vi "AssertValueByArrayName.vi"(0 "VI Reference In":refnum<vi>, 1 "Test Label":string, 2 "delimiter (>>)":string=">>", 3 "Assert Only? (F)":bool, 5 "Control Path":string, 7 "Focus Item Names":string[](array[string]), 11 "Error In":errorcluster, 12 "Assert Interval(10 ms)":u32=10, 13 "Timeout(5 sec)":dbl=5.0) -> (4 "VI Reference Out":refnum<vi>, 6 "Asserted Value":string[](array[string]), 15 "Error Out":errorcluster)   [LabVIEW 2016, in "Drona.lvlib" / "AssertControlValue.lvlib" / "AssertMCListbox.lvlib"]
doc: "Asserts if the focus item first column names of multi-select listbox control are equal.\n\nThe input control name is given as a string, incase of the path, use delimiters in between the path.\nThis VI gets the control value until the value is equal to the input value."
uses:
  AssertMCListbox.lvlib
  Get/GetControlRef/GetControlRefByPath.vi
  <userlib>/_OpenG.lib/array/array.llb/Index 1D Array Elements (String)__ogtk.vi
  <vilib>/addons/_JKI Toolkits/Caraya/classes/Assert/Assert Equal Value_Variant.vi
  <vilib>/Utility/error.llb/Error Cluster From Error Code.vi
  <vilib>/ErrorRing/Error Ring.xnode
  <vilib>/addons/_JKI Toolkits/Caraya/classes/Assert/Assert.lvclass
  Get/GetControlRef/GetControlRef.lvlib
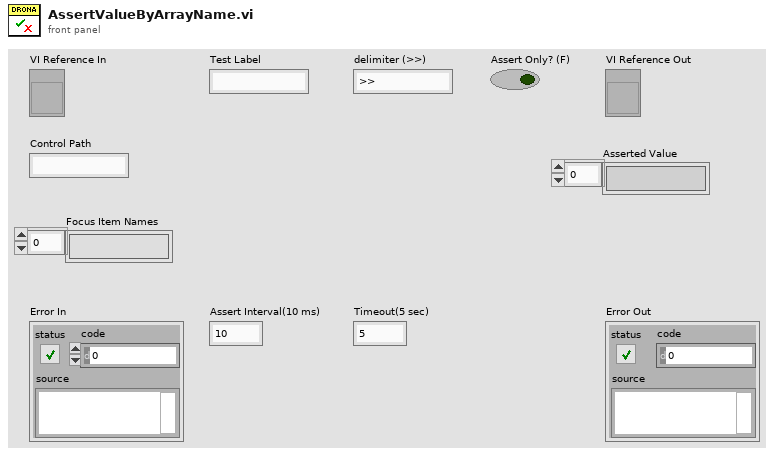
[diagram p1: front panel]
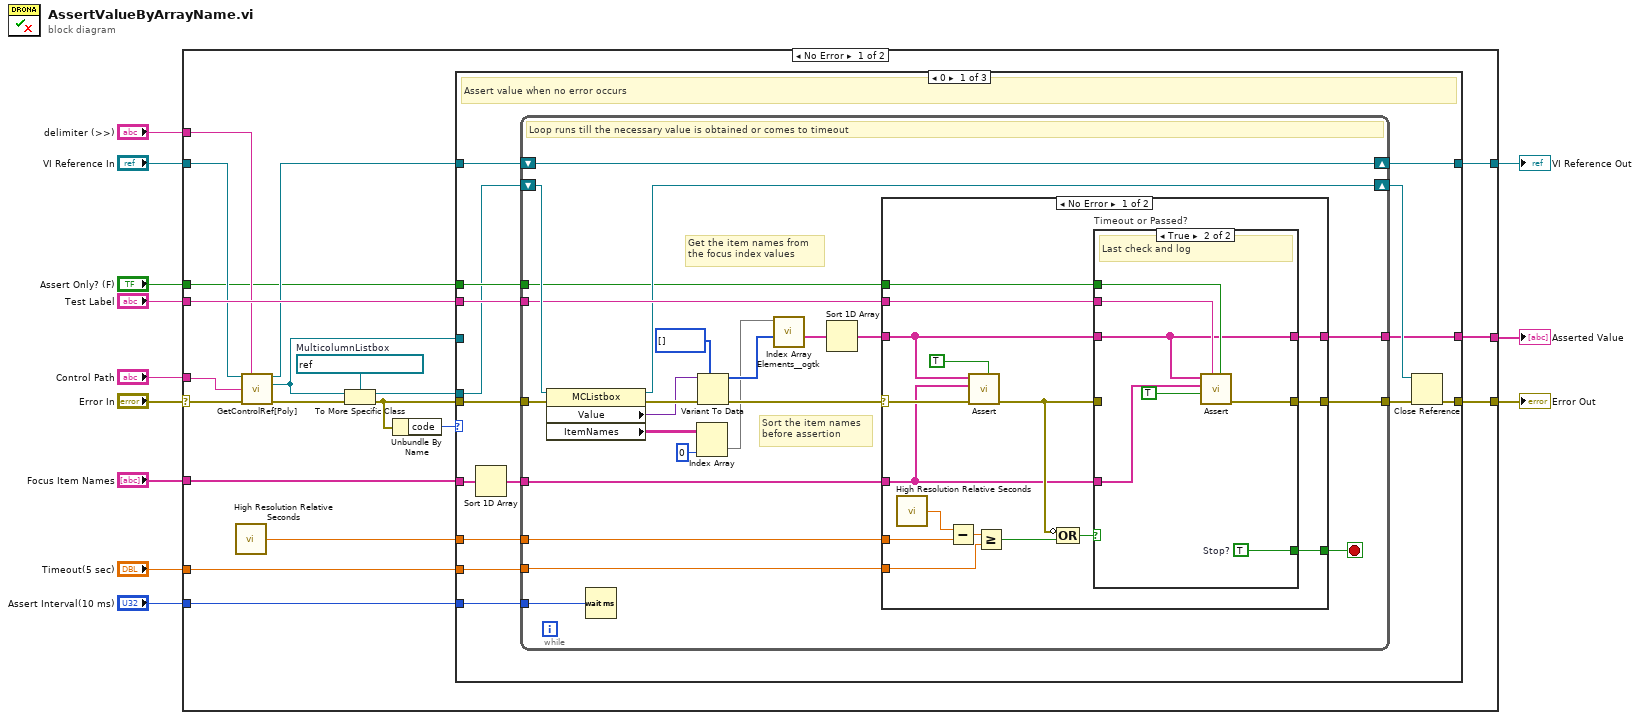
[diagram p0: block diagram]
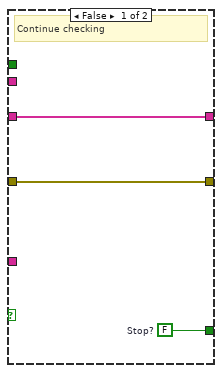
[diagram p2: hidden frame]
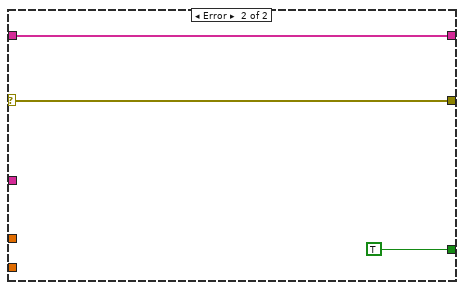
[diagram p3: hidden frame]
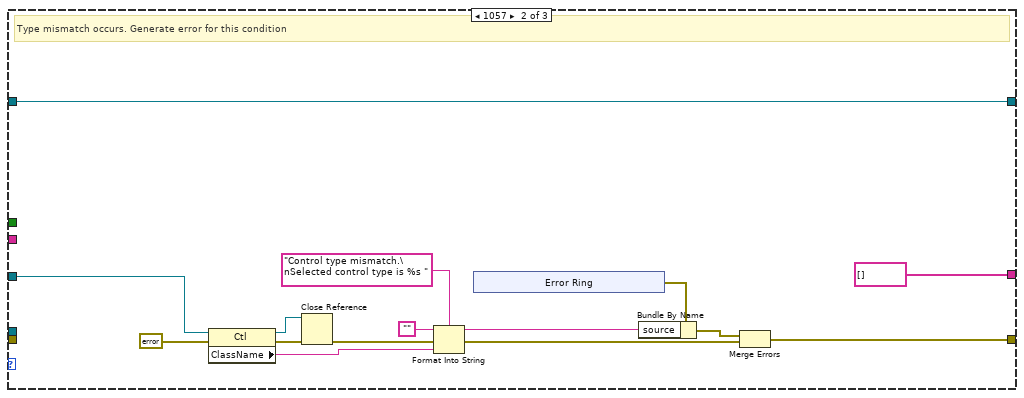
[diagram p4: hidden frame]
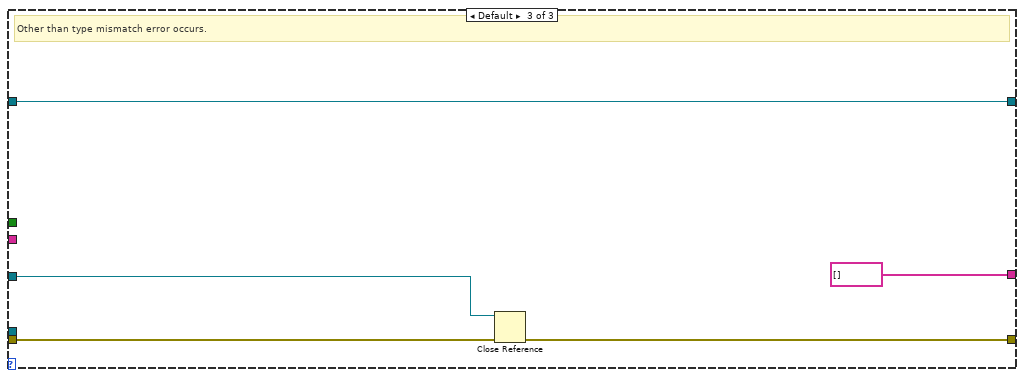
[diagram p5: hidden frame]
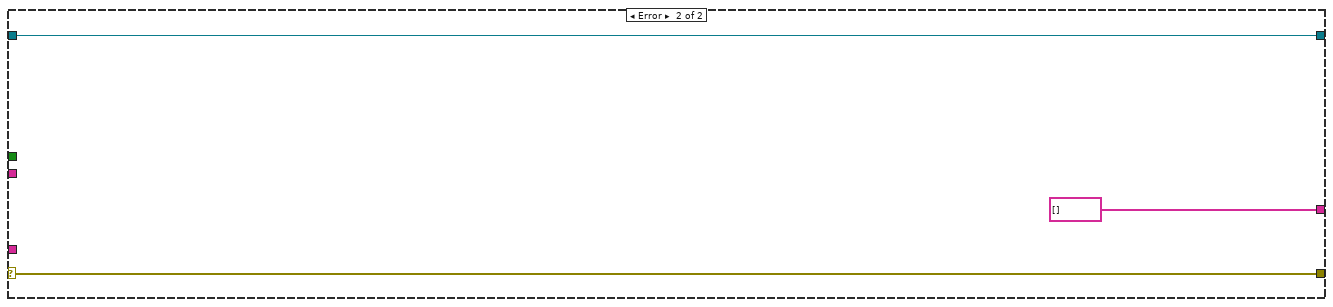
[diagram p6: hidden frame]
diagram:
  n1 = case shown="No Error" "Error In" {
    selector: "Error In" -> [w28 w127]
    tunnel: "Timeout(5 sec)" -> [w32 _]
    tunnel: [w31 w126] -> w11
    tunnel: [w22 w127] -> w10
    tunnel: "Assert Interval(10 ms)" -> [w30 _]
    tunnel: "Test Label" -> [w29 _]
    tunnel: "VI Reference In" -> [w27 w126]
    tunnel: "Control Path" -> [w26 _]
    tunnel: "delimiter (>>)" -> [w21 _]
    tunnel: "Assert Only? (F)" -> [w20 _]
    tunnel: [w19 string[] []] -> w2
    tunnel: "Focus Item Names" -> [w16 _]
    frame No Error {
      w18 = refnum<vi> refnum  # MulticolumnListbox
      n2 = call <vilib>:"High Resolution Relative Seconds.vi"() -> ("relative seconds"=w25:dbl)
      n3 = call-poly "GetControlRef[Poly].vi"("VI Reference In"=w27, "delimiter (>>)"=w21, "Control Path"=w26, "error In"=w28) -> ("VI Reference Out"=w23:refnum<vi>, "Ctl Refnum"=w13:refnum<vi>, "error out"=w24:errorcluster)  [unwired: 9 in]
      n4 = To More Specific Class(target class=w18, reference=w13, error in=w24) -> (specific class reference=w17:refnum<vi>, error out=w15:errorcluster)
      n5 = Unbundle By Name(w15) -> ("code"=w14:i32)
      n6 = case shown="0" w14 {
        tunnel: w32 -> [w47 _ _]
        tunnel: [w46 w100 w123] -> w31
        tunnel: w30 -> [w44 _ _]
        tunnel: w29 -> [w43 _ _]
        tunnel: w25 -> [w42 _ _]
        tunnel: w23 -> [w41 w100 w123]
        tunnel: [w40 w103 w121] -> w22
        tunnel: w20 -> [w38 _ _]
        tunnel: [w33 string[] [] string[] []] -> w19
        tunnel: w15 -> [w37 _ w124]
        tunnel: w17 -> [w36 _ _]
        tunnel: w16 -> [w35 _ _]
        tunnel: w13 -> [_ w102 w120]
        frame 0 {
          # "Assert value when no error occurs"
          n7 = Sort 1D Array(array=w35) -> (sorted array=w34:string[])
          n8 = while {
            tunnel: w47 -> [w69]
            tunnel: w42 -> [w70]
            tunnel: w37 -> [w64]
            tunnel: [w67] -> w45
            tunnel: w44 -> [w65]
            tunnel: w43 -> [w61]
            shift-right: [w62] -> w46
            shift-left: w41 -> [w62]
            shift-right: [w60] -> w39
            shift-left: w36 -> [w63]
            tunnel: w38 -> [w59]
            tunnel: [w58] -> w33
            tunnel: w34 -> [w54]
            stop <- w68 stop-if-true
            # "Sort the item names \nbefore assertion"
            # "Get the item names from \nthe focus index values"
            # "Loop runs till the necessary value is obtained or comes to timeout"
            n9 = property on="Property Node" class="MCListbox"(reference=w63, error in=w64) -> (reference out=w60:refnum<vi>, error out=w66:errorcluster, "Value"=w56:variant, "ItemNames"=w50:string[][])
            n10 = Wait (ms)(milliseconds to wait=w65) -> ()  [unwired: 1 out]
            n11 = Index Array(array=w50, index (col)=0 ("disabled index (col)")) -> (element=w48:string[])  [unwired: 1 in]
            n12 = Variant To Data(error in=w66, type=i32[] [], Variant=w56) -> (data=w52:i32[], error out=w57:errorcluster)
            n13 = call-poly <userlib>:"Index Array Elements__ogtk.vi"("indices"=w52, "array"=w48) -> ("elements"=w51:string[])  [unwired: 9 in]
            n14 = Sort 1D Array(array=w51) -> (sorted array=w53:string[])
            n15 = case shown="No Error" w57 {
              selector: w57 -> [w82 w99]
              tunnel: w70 -> [w86 _]
              tunnel: w69 -> [w83 _]
              tunnel: [w73 TRUE] -> w68
              tunnel: [w74 w99] -> w67
              tunnel: w54 -> [w75 _]
              tunnel: w53 -> [w76 w97]
              tunnel: w61 -> [w81 _]
              tunnel: w59 -> [w72 _]
              tunnel: [w71 w97] -> w58
              frame No Error {
                n16 = call <vilib>:"High Resolution Relative Seconds.vi"() -> ("relative seconds"=w85:dbl)
                n17 = Subtract(x=w85, y=w86) -> (x-y=w84:dbl)
                n18 = call-poly <vilib>:"Assert.vi"("Assert Only? (F)"=TRUE, "error in (no error)"=w82, "Y"=w75, "X"=w76) -> ("error out"=w79:errorcluster)  [unwired: 6 in, 1 out]
                n19 = Greater Or Equal?(x=w84, y=w83) -> (x >= y?=w80:bool)
                n20 = Compound Arithmetic op=OR(invert w79, w80) -> (w78:bool)
                n21 = case "Timeout or Passed?" shown="True" w78 {
                  tunnel: w79 -> [w89 _]
                  tunnel: w75 -> [_ w91]
                  tunnel: w76 -> [w87 w92]
                  tunnel: w81 -> [_ w96]
                  tunnel: [w89 w95] -> w74
                  tunnel: [w88 w94] -> w73
                  tunnel: w72 -> [_ w93]
                  tunnel: [w87 w92] -> w71
                  frame False {
                    w88 = FALSE  # Stop?
                    # "Continue checking"
                  }
                  frame True {
                    w94 = TRUE  # Stop?
                    # "Last check and log"
                    n22 = call-poly <vilib>:"Assert.vi"("Assert Only? (F)"=w93, "Label"=w96, "Register with caller test (F)"=TRUE, "Y"=w91, "X"=w92) -> ("error out"=w95:errorcluster)  [unwired: 5 in, 1 out]
                  }
                }
              }
              frame Error {
              }
            }
          }
          n23 = Close Reference(reference=w39, error in (no error)=w45) -> (error out=w40:errorcluster)
        }
        frame 1057 {
          # "Type mismatch occurs. Generate error for this condition"
          n24 = property class="Ctl"(reference=w102, error in=errorcluster {"status"=FALSE, "code"=0, "source"=""} ("error out")) -> (reference out=w104:refnum<vi>, error out=w114:errorcluster, "ClassName"=w111:string)
          n25 = Close Reference(reference=w104, error in (no error)=w114) -> (error out=w105:errorcluster)
          n26 = Format Into String(format string="Control type mismatch.\nSelected control type is %s ", initial string="", error in=w105, w111) -> (resulting string=w108:string, error out=w106:errorcluster)
          n27 = xnode "Error Ring"() -> ("error out"=w109:errorcluster)
          n28 = Bundle By Name(cluster=w109, "source"=w108) -> (w107:errorcluster)
          n29 = Merge Errors(w107, w106) -> (w103:errorcluster)
        }
        frame Default {
          # "Other than type mismatch error occurs."
          n30 = Close Reference(reference=w120, error in (no error)=w124) -> (error out=w121:errorcluster)
        }
      }
    }
    frame Error {
    }
  }
  "Error Out" <- w10
  "VI Reference Out" <- w11
  "Asserted Value" <- w2
